vi "scopeGUI.vi"() -> ()   [LabVIEW 2023]
panel:
  in  "Extract button":bool
  out "standard output":string
  in  "CH2 units":string(combo)
  in  "∆V CH2":string
  in  "CH1 units":string(combo)
  in  "∆V CH1":string
  in  "t units":string(combo)
  in  "∆t":string
  out "CH1":bool
  out "CH2":bool
  in  "Select channel":bool
  in  "Last file":dbl=1.0 min=1.0 max=20.0
  in  "First file":dbl=1.0 min=1.0 max=20.0 step=1.0
  in  "Output path":path
  in  "Input path":path
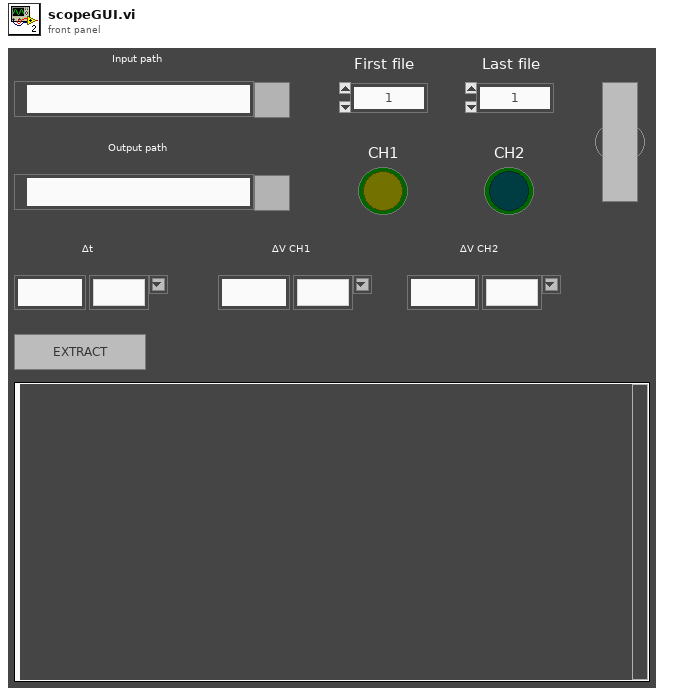
[diagram p1: front panel]
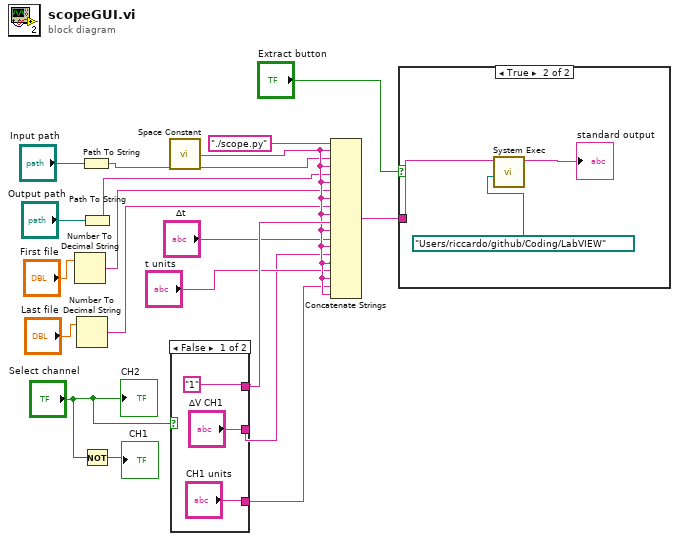
[diagram p0: block diagram]
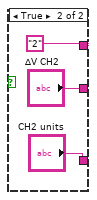
[diagram p3: hidden frame]
diagram:
  n1 = Number To Decimal String(number="First file") -> (decimal integer string=w13:string)  [unwired: 1 in]
  n2 = Number To Decimal String(number="Last file") -> (decimal integer string=w14:string)  [unwired: 1 in]
  n3 = Path To String(path="Input path") -> (string=w9:string)
  n4 = Path To String(path="Output path") -> (string=w10:string)
  n5 = Not(x="Select channel") -> (.not. x?=→"CH1":bool)
  n6 = call <vilib>:"Space Constant.vi"() -> ("String"=w18:string)
  n7 = case shown="False" "Select channel" {
    tunnel: ["1" "2"] -> w19
    tunnel: ["∆V CH1" "∆V CH2"] -> w2
    tunnel: ["CH1 units" "CH2 units"] -> w17
    frame False {
    }
    frame True {
    }
  }
  n8 = Concatenate Strings("./scope.py", w18, w9, w18, w10, w18, w13, w18, w14, w18, w19, w18, "∆t", w18, w2, w18, "t units", w18, w17, w18) -> (w8:string)
  n9 = case shown="True" "Extract button" {
    tunnel: w8 -> [_ w28]
    frame False {
    }
    frame True {
      n10 = call <vilib>:"System Exec.vi"("working directory"=path "/Users/riccardo/github/Coding/LabVIEW", "command line"=w28) -> ("standard output"=→"standard output":string)  [unwired: 6 in, 3 out]
    }
  }
  "CH2" <- "Select channel"
